vi "Read Rank.vi"(8 "error in (no error)":errorcluster, 11 "SG 54GHz Path Group in":refnum<class "SG 54GHz Path Group.lvclass">) -> (0 "error out":errorcluster, 2 "Rank":dbl, 3 "SG 54GHz Path Group out":refnum<class "SG 54GHz Path Group.lvclass">)   [LabVIEW 2023, in "RFFixtureCharact.RMM.lvlib" / "SG 54GHz Path Group.lvclass"]
uses:
  SG 54GHz Path Group.lvclass
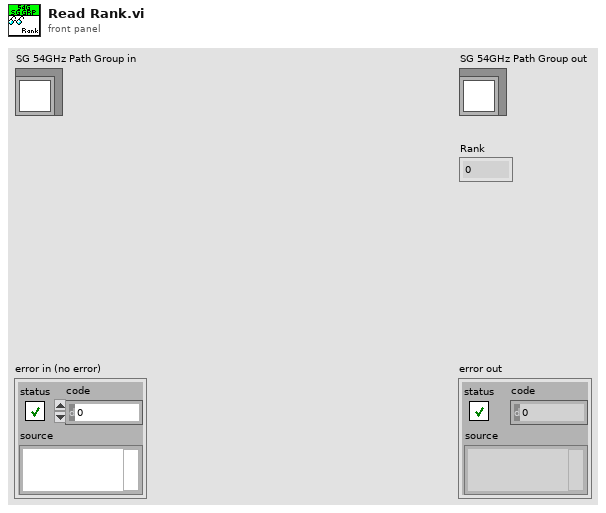
[diagram p1: front panel]
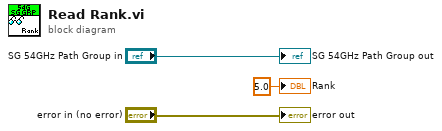
[diagram p0: block diagram]
diagram:
  "error out" <- "error in (no error)"
  "SG 54GHz Path Group out" <- "SG 54GHz Path Group in"
  "Rank" <- 5.0 ("Rank")
